vi "Get Distance Readings.vi"(8 "error in (no error)":errorcluster, 11 "Mouse in":refnum<class "Mouse.lvclass">) -> (0 "error out":errorcluster, 2 "Distances":T1, 3 "Mouse out":refnum<class "Mouse.lvclass">)   [LabVIEW 2020, in "Maze.lvlib" / "Mouse.lvclass"]
doc: "This property returns the current distance to walls in each direction relative to where the mouse is facing. For instance if there is a wall directly in front of where the mouse is facing, the Forward distance will be 0. Trying to move forward while the Forward distance is 0 will result in a wall crash and end the run so try and make sure you're protecting your noggin."
uses:
  Mouse.lvclass
  Distances.ctl
  Mouse.lvclass/Mouse.ctl
  Maze.lvlib
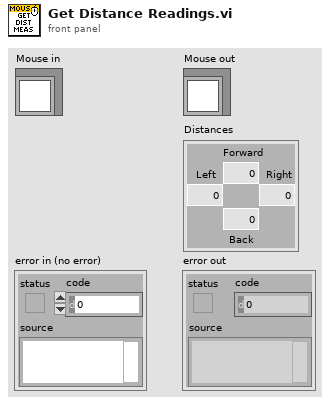
[diagram p1: front panel]
types:
  T1 = typedef "Maze.lvlib/Distances.ctl" = cluster{"Forward":i32, "Back":i32, "Left":i32, "Right":i32}
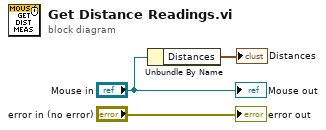
[diagram p0: block diagram]
diagram:
  n1 = Unbundle By Name("Mouse in") -> ("Distances"=→"Distances":T1)
  "error out" <- "error in (no error)"
  "Mouse out" <- "Mouse in"
